vi "90 Names.vi"() -> ()   [LabVIEW 2018]
uses:
  <vilib>/Rock Robotics/WPI/Joystick/WPI_JoystickDeviceEnum.ctl
  <vilib>/Rock Robotics/SystemInterfaces/DIO/FPGA_DIOPWMChannel.ctl
  <vilib>/Rock Robotics/SystemInterfaces/DIO/FPGA_DIOChannel.ctl
  <vilib>/Rock Robotics/WPI/MotorControl/WPI_MotorControlOpen Talon.vi
  <vilib>/Rock Robotics/WPI/Switch/WPI_SwitchOpenLimit.vi
  <vilib>/Rock Robotics/WPI/MotorControl/WPI_MotorControlOpen SPARK.vi
  <vilib>/Rock Robotics/WPI/Utilities/WPI_GetSetVariantRefNum.vi
panel:
  in  "Wrist Out Speed":dbl=0.5
  in  "Wrist In Speed":dbl=0.5
  out "POVs":i16[](array[numeric])
  out "Buttons":bool[](array[boolean])
  out "Axes":dbl[](array[numeric])
  in  "stop":bool
  out "Output":dbl(slide) scale=0.0..1.0
  out "Joystick X":dbl(slide) scale=1.0..-1.0
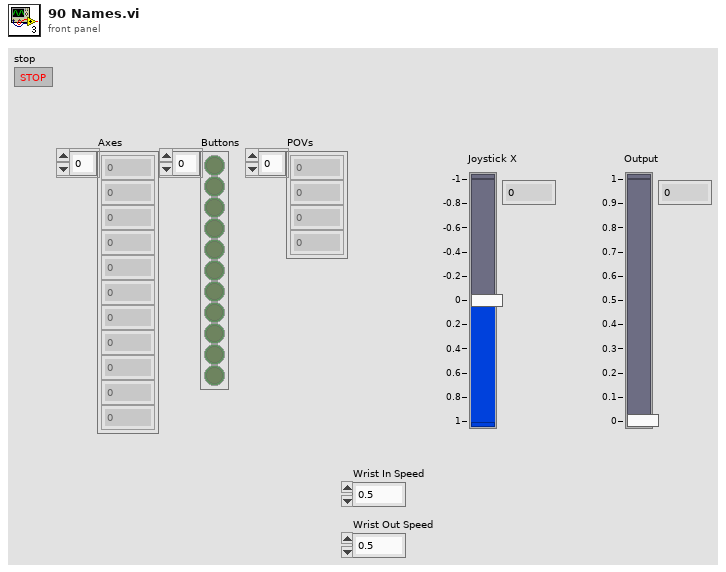
[diagram p1: front panel]
types:
  T1 = typedef "FPGA_DIOPWMChannel.ctl" = enum8{"PWM 0", "PWM 1", "PWM 2", "PWM 3", "PWM 4", "PWM 5", "PWM 6", "PWM 7", "PWM 8", "PWM 9", "PWM MXP 0", "PWM MXP 1", "PWM MXP 2", "PWM MXP 3", "PWM MXP 4", "PWM MXP 5", "PWM MXP 6", "PWM MXP 7", "PWM MXP 8", "PWM MXP 9", "Invalid"}
  T2 = typedef "FPGA_DIOChannel.ctl" = enum8{"DIO 0", "DIO 1", "DIO 2", "DIO 3", "DIO 4", "DIO 5", "DIO 6", "DIO 7", "DIO 8", "DIO 9", "DIO MXP 0", "DIO MXP 1", "DIO MXP 2", "DIO MXP 3", "DIO MXP 4", "DIO MXP 5", "DIO MXP 6", "DIO MXP 7", "DIO MXP 8", "DIO MXP 9", "DIO MXP 10", "DIO MXP 11", "DIO MXP 12", "DIO MXP 13", "DIO MXP 14", "DIO MXP 15", "SPI Port CS1", "SPI Port CS2", "SPI Port CS3", "SPI Port MISO", "SPI Port MOSI", "Invalid"}
  T3 = typedef "WPI_JoystickDeviceEnum.ctl" = enum16{"USB 0", "USB 1", "USB 2", "USB 3", "USB 4", "USB 5"}
  T4 = typedef "WPI_MotorControlDeviceRef.ctl" = cluster{"DeviceStatus":errorcluster, "Type":T5, "PWM":cluster{"PWM Channel":T1, "DeadBand":T6}, "CAN":cluster{"Device Number":u8, "SetOutput VI Ref":variant, "GetOutput VI Ref":variant, "Enable VI Ref":variant, "Disable VI Ref":variant, "Data":variant}, "Invert":bool, "DIO PWM":cluster{"PWM \"Enable\" Channel":T1, "DIOChannel":T2, "PWM Rate":dbl}}
  T5 = typedef "WPI_MotorControlType.ctl" = enum16{"PWM", "CAN", "DIO PWM"}
  T6 = typedef "WPI_PWMDeadband.ctl" = cluster{"Name":string, "maxPositivePwm":i32, "minPositivePwm":i32, "centerPwm":i32, "maxNegativePwm":i32, "minNegativePwm":i32, "angularRange":u16}
  T7 = typedef "WPI_JoystickDevRef.ctl" = cluster{"Device":T3}
  T8 = typedef "WPI_SwitchDevRef.ctl" = cluster{"DevStatus":errorcluster, "DIO Channel":T2, "CntIndex":T9, "Normally Closed":bool}
  T9 = typedef "FPGA_CounterCtrSystemIndex.ctl" = enum8{"Ctr 0", "Ctr 1", "Ctr 2", "Ctr 3", "Ctr 4", "Ctr 5", "Ctr 6", "Ctr 7", "Invalid"}
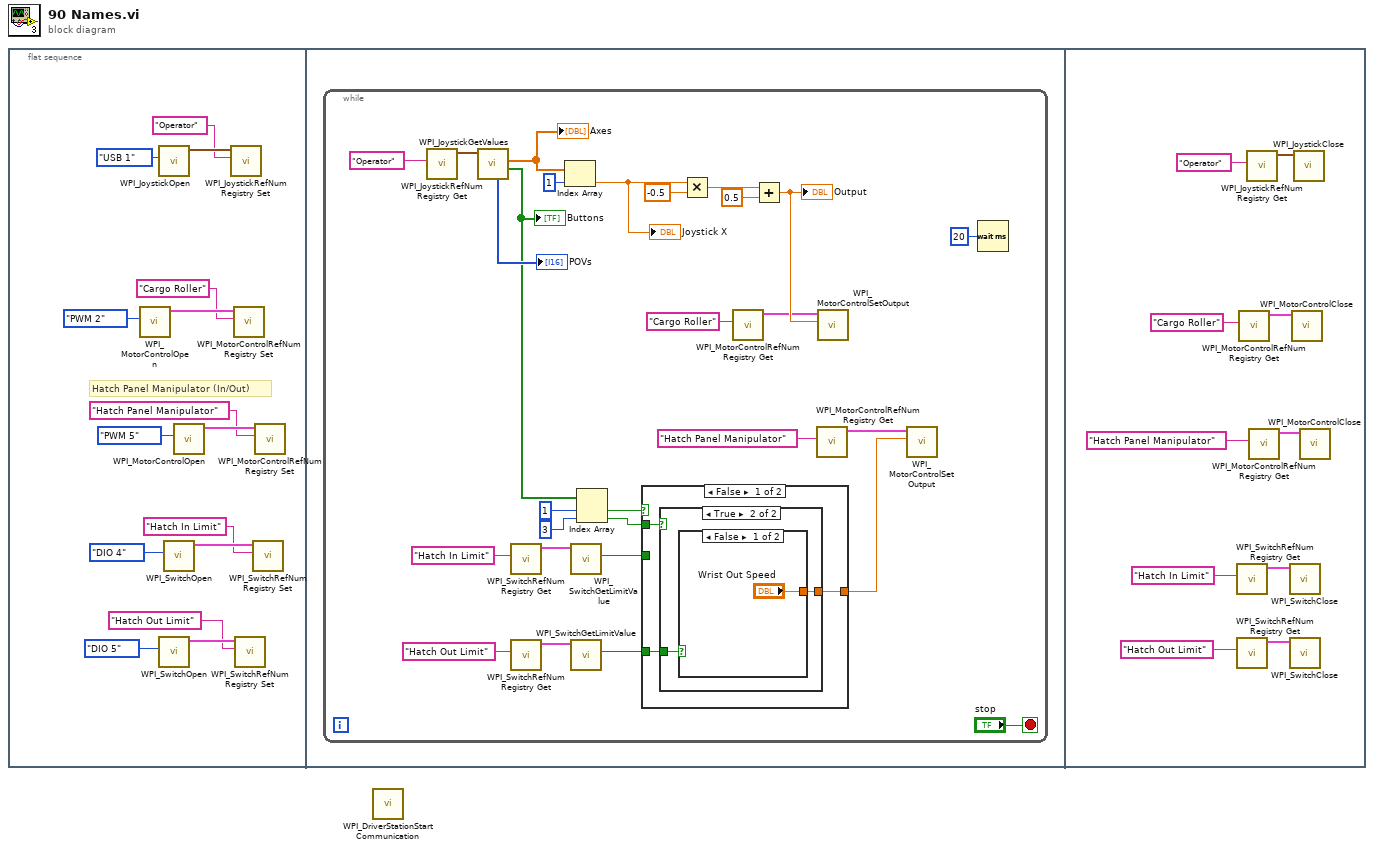
[diagram p0: block diagram]
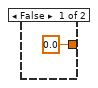
[diagram p2: hidden frame]
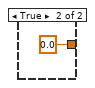
[diagram p3: hidden frame]
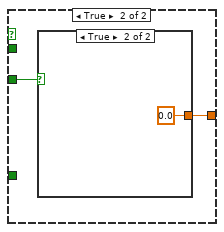
[diagram p4: hidden frame]
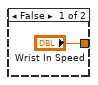
[diagram p5: hidden frame]
diagram:
  n1 = flat-sequence {
    frame #0 {
      # "Hatch Panel Manipulator (In/Out)"
      n2 = call-poly <vilib>:"WPI_MotorControlOpen.vi"("PWM Channel"=FPGA_DIOPWMChannel."PWM 2") -> ("MotorControlDeviceRef"=w8:T4)  [unwired: 9 in, 1 out]
      n3 = call <vilib>:"WPI_JoystickOpen.vi"("JoystickDevice"=WPI_JoystickDeviceEnum."USB 1") -> ("JoystickDevRef"=w10:T7)  [unwired: 10 in]
      n4 = call-poly <vilib>:"WPI_SwitchOpen.vi"("DIO Channel"=FPGA_DIOChannel."DIO 5") -> ("SwitchDevRef"=w2:T8)  [unwired: 9 in, 1 out]
      n5 = call-poly <vilib>:"WPI_SwitchOpen.vi"("DIO Channel"=FPGA_DIOChannel."DIO 4") -> ("SwitchDevRef"=w4:T8)  [unwired: 9 in, 1 out]
      n6 = call-poly <vilib>:"WPI_MotorControlOpen.vi"("PWM Channel"=FPGA_DIOPWMChannel."PWM 5") -> ("MotorControlDeviceRef"=w6:T4)  [unwired: 9 in, 1 out]
      n7 = call <vilib>:"WPI_JoystickRefNum Registry Set.vi"("refnum name"="Operator", "JoystickDevRef"=w10) -> ()  [unwired: 8 in, 2 out]
      n8 = call <vilib>:"WPI_MotorControlRefNum Registry Set.vi"("refnum name"="Cargo Roller", "MotorControlDevRef"=w8) -> ()  [unwired: 8 in, 2 out]
      n9 = call <vilib>:"WPI_SwitchRefNum Registry Set.vi"("refnum name"="Hatch Out Limit", "SwitchDevRef"=w2) -> ()  [unwired: 8 in, 2 out]
      n10 = call <vilib>:"WPI_SwitchRefNum Registry Set.vi"("refnum name"="Hatch In Limit", "SwitchDevRef"=w4) -> ()  [unwired: 8 in, 2 out]
      n11 = call <vilib>:"WPI_MotorControlRefNum Registry Set.vi"("refnum name"="Hatch Panel Manipulator", "MotorControlDevRef"=w6) -> ()  [unwired: 8 in, 2 out]
    }
    frame #1 {
      n12 = while {
        stop <- "stop" stop-if-true
        n13 = call <vilib>:"WPI_JoystickRefNum Registry Get.vi"("refnum name"="Operator") -> ("JoystickDevRef"=w17:T7)  [unwired: 9 in, 1 out]
        n14 = call <vilib>:"WPI_JoystickGetValues.vi"("JoystickDevRef"=w17) -> ("Buttons"=w33:bool[], "Axes"=w38:dbl[], "POVs"=→"POVs":i16[])  [unwired: 6 in, 2 out]
        "Axes" <- w38
        "Buttons" <- w33
        n15 = call <vilib>:"WPI_SwitchRefNum Registry Get.vi"("refnum name"="Hatch In Limit") -> ("SwitchDevRef"=w25:T8)  [unwired: 9 in, 1 out]
        n16 = call <vilib>:"WPI_SwitchRefNum Registry Get.vi"("refnum name"="Hatch Out Limit") -> ("SwitchDevRef"=w24:T8)  [unwired: 9 in, 1 out]
        n17 = Index Array(array=w38, index=1) -> (element=w36:dbl)
        "Joystick X" <- w36
        n18 = call <vilib>:"WPI_SwitchGetLimitValue.vi"("SwitchDevRef"=w25) -> ("Switch Pressed"=w29:bool)  [unwired: 8 in, 2 out]
        n19 = call <vilib>:"WPI_SwitchGetLimitValue.vi"("SwitchDevRef"=w24) -> ("Switch Pressed"=w26:bool)  [unwired: 8 in, 2 out]
        n20 = Index Array(array=w33, index #1=1 ("index"), index #2=3 ("index")) -> (element #1=w30:bool, element #2=w27:bool)
        n21 = case shown="False" w30 {
          tunnel: w29 -> [_ w53]
          tunnel: [w44 w52] -> w28
          tunnel: w27 -> [w46 _]
          tunnel: w26 -> [w45 _]
          frame False {
            n22 = case shown="True" w46 {
              tunnel: w45 -> [_ w49]
              tunnel: [0.0 ("Wrist Out Speed") w48] -> w44
              frame False {
              }
              frame True {
                n23 = case shown="False" w49 {
                  tunnel: ["Wrist Out Speed" 0.0] -> w48
                  frame False {
                  }
                  frame True {
                  }
                }
              }
            }
          }
          frame True {
            n24 = case shown="True" w53 {
              tunnel: ["Wrist In Speed" 0.0] -> w52
              frame False {
              }
              frame True {
              }
            }
          }
        }
        n25 = Multiply(x=w36, y=-0.5) -> (x*y=w40:dbl)
        n26 = call <vilib>:"WPI_MotorControlRefNum Registry Get.vi"("refnum name"="Cargo Roller") -> ("MotorControlDevRef"=w21:T4)  [unwired: 9 in, 1 out]
        n27 = Add(x=w40, y=0.5) -> (x+y=w34:dbl)
        "Output" <- w34
        n28 = call <vilib>:"WPI_MotorControlRefNum Registry Get.vi"("refnum name"="Hatch Panel Manipulator") -> ("MotorControlDevRef"=w20:T4)  [unwired: 9 in, 1 out]
        n29 = call <vilib>:"WPI_MotorControlSetOutput.vi"("Output"=w34, "MotorControlDevRef"=w21) -> ()  [unwired: 7 in, 3 out]
        n30 = call <vilib>:"WPI_MotorControlSetOutput.vi"("Output"=w28, "MotorControlDevRef"=w20) -> ()  [unwired: 7 in, 3 out]
        n31 = Wait (ms)(milliseconds to wait=u32 20) -> ()  [unwired: 1 out]
      }
    }
    frame #2 {
      n32 = call <vilib>:"WPI_SwitchRefNum Registry Get.vi"("refnum name"="Hatch In Limit") -> ("SwitchDevRef"=w64:T8)  [unwired: 9 in, 1 out]
      n33 = call <vilib>:"WPI_SwitchRefNum Registry Get.vi"("refnum name"="Hatch Out Limit") -> ("SwitchDevRef"=w65:T8)  [unwired: 9 in, 1 out]
      n34 = call <vilib>:"WPI_MotorControlRefNum Registry Get.vi"("refnum name"="Cargo Roller") -> ("MotorControlDevRef"=w62:T4)  [unwired: 9 in, 1 out]
      n35 = call <vilib>:"WPI_JoystickRefNum Registry Get.vi"("refnum name"="Operator") -> ("JoystickDevRef"=w61:T7)  [unwired: 9 in, 1 out]
      n36 = call <vilib>:"WPI_MotorControlRefNum Registry Get.vi"("refnum name"="Hatch Panel Manipulator") -> ("MotorControlDevRef"=w63:T4)  [unwired: 9 in, 1 out]
      n37 = call <vilib>:"WPI_SwitchClose.vi"("SwitchDevRef"=w64) -> ()  [unwired: 10 in, 1 out]
      n38 = call <vilib>:"WPI_SwitchClose.vi"("SwitchDevRef"=w65) -> ()  [unwired: 10 in, 1 out]
      n39 = call <vilib>:"WPI_MotorControlClose.vi"("MotorControlDevRef"=w62) -> ()  [unwired: 10 in, 1 out]
      n40 = call <vilib>:"WPI_JoystickClose.vi"("JoystickDevRef"=w61) -> ()  [unwired: 11 in]
      n41 = call <vilib>:"WPI_MotorControlClose.vi"("MotorControlDevRef"=w63) -> ()  [unwired: 10 in, 1 out]
    }
  }
  n42 = call <vilib>:"WPI_DriverStationStart Communication.vi"() -> ()  [unwired: 12 in]
